vi "Write SHV Enabled.vi"(8 "error in (no error)":errorcluster, 10 "Enabled (F)":bool, 11 "Stepper in":refnum<class "Stepper.lvclass">) -> (0 "error out":errorcluster, 3 "Stepper out":refnum<class "Stepper.lvclass">)   [LabVIEW 2015, in "Stepper.lvclass"]
uses:
  Stepper.lvclass
  Stepper.lvclass/Stepper.ctl
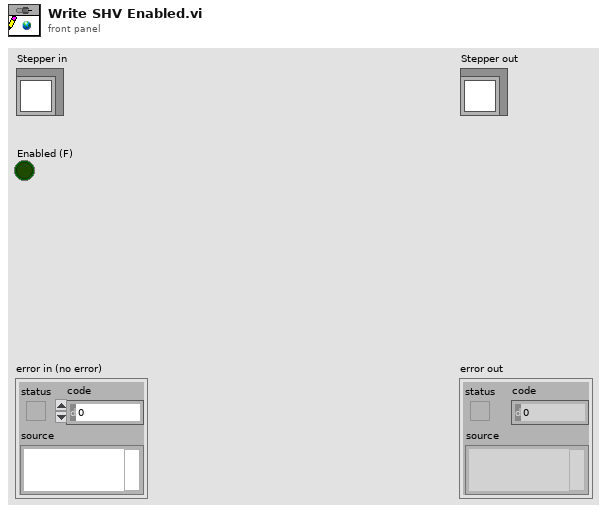
[diagram p1: front panel]
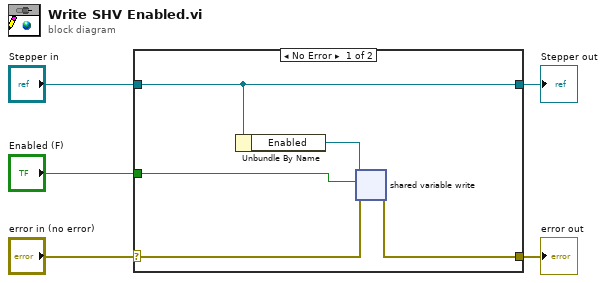
[diagram p0: block diagram]
diagram:
  n1 = case shown="No Error" "error in (no error)" {
    selector: "error in (no error)" -> [w10 w11]
    tunnel: [w9 w11] -> w4
    tunnel: [w7 w12] -> w2
    tunnel: "Stepper in" -> [w7 w12]
    tunnel: "Enabled (F)" -> [w8 _]
    frame No Error {
      n2 = Unbundle By Name(w7) -> ("Enabled"=w6:refnum<k21>)
      n3 = shared-variable-write(w6, w10, w8) -> (w9:errorcluster)  [unwired: 1 out]
    }
    frame Error {
    }
  }
  "error out" <- w4
  "Stepper out" <- w2
